vi "getGridElements.vi"(8 "error in (no error)":errorcluster, 11 "CategoryList in":refnum<class "CategoryList.lvclass">) -> (0 "error out":errorcluster, 2 "Table Interface":string[][](array[string]), 3 "CategoryList out":refnum<class "CategoryList.lvclass">)   [LabVIEW 2020, in "CategoryList.lvclass"]
uses:
  CategoryList.lvclass
  CategoryList.lvclass/CategoryList.ctl
  Category/Category.lvclass
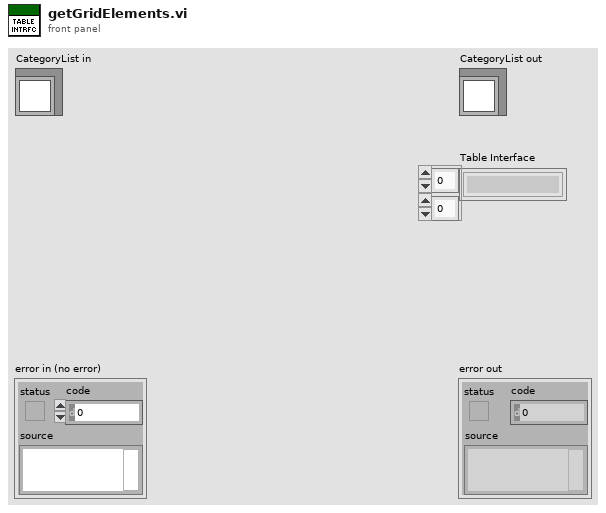
[diagram p1: front panel]
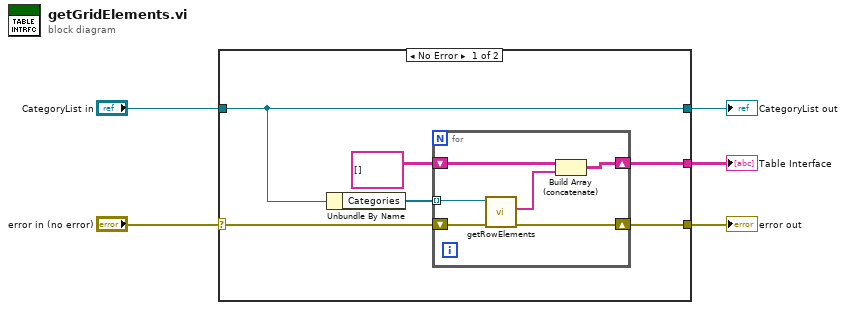
[diagram p0: block diagram]
diagram:
  n1 = case shown="No Error" "error in (no error)" {
    selector: "error in (no error)" -> [w9 w19]
    tunnel: [w8 w19] -> w4
    tunnel: [w11 w18] -> w2
    tunnel: "CategoryList in" -> [w11 w18]
    tunnel: [w6 _] -> w1
    frame No Error {
      n2 = Unbundle By Name(w11) -> ("Categories"=w10:refnum<class "Category.lvclass">[])
      n3 = for {
        shift-right: [w15] -> w8
        shift-left: w9 -> [w16]
        tunnel: w10 -> [w17] mode=indexing
        shift-right: [w12] -> w6
        shift-left: string[][] [] ("String Array") -> [w14]
        n4 = call-dynamic "getRowElements.vi"("error in (no error)"=w16, "Category in"=w17) -> ("error out"=w15:errorcluster, "Row Interface"=w13:string[])  [unwired: 7 in, 1 out]
        n5 = Build Array (concatenate)(w14, w13) -> (w12:string[][])
      }
    }
    frame Error {
    }
  }
  "error out" <- w4
  "CategoryList out" <- w2
  "Table Interface" <- w1
